vi "SeqMgr.Set Test Stop Criteria.vi"(8 "error in":errorcluster, 9 "Stop on Error":bool=TRUE, 10 "Stop on Fail":bool, 11 "SeqMgr in":refnum<class "SeqMgr.lvclass">) -> (0 "error out":errorcluster, 3 "SeqMgr out":refnum<class "SeqMgr.lvclass">)   [LabVIEW 2024, in "EQMF.lvlib" / "SeqMgr.lvlib" / "SeqMgr.lvclass"]
uses:
  SeqMgr.lvclass
  SeqMgr.lvclass/SeqMgr.ctl
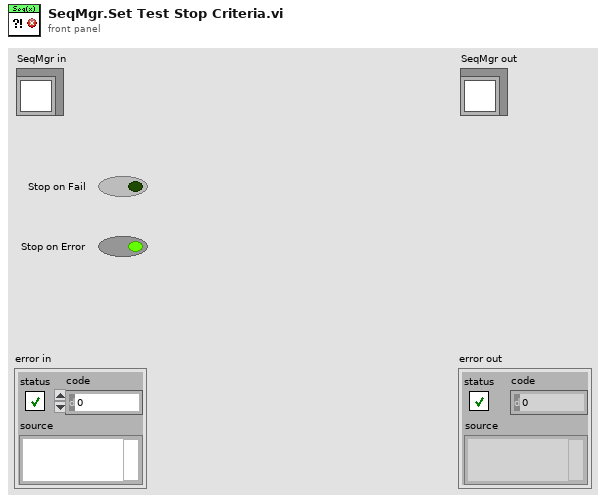
[diagram p1: front panel]
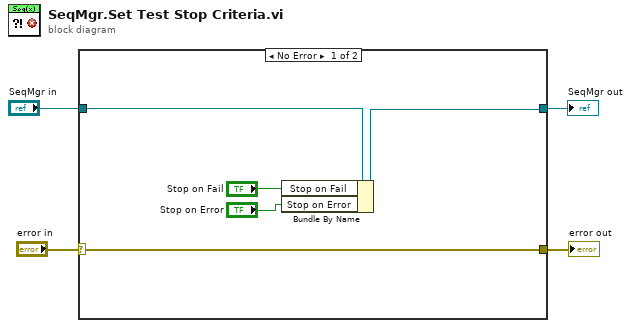
[diagram p0: block diagram]
diagram:
  n1 = case shown="No Error" "error in" {
    selector: "error in" -> [w9 w11]
    tunnel: [w9 w11] -> w3
    tunnel: [w7 w10] -> w1
    tunnel: "SeqMgr in" -> [w8 w10]
    frame No Error {
      n2 = Bundle By Name(cluster=w8, "Stop on Fail"="Stop on Fail", "Stop on Error"="Stop on Error") -> (w7:refnum<class "SeqMgr.lvclass">)
    }
    frame Error {
    }
  }
  "error out" <- w3
  "SeqMgr out" <- w1
